vi "Handle getAll.vi"(8 "error in (no error)":errorcluster, 11 "Instrument.Transport in":refnum<class "Inst.Transport.lvclass">) -> (0 "error out":errorcluster, 2 "getAll":variant, 3 "Instrument.Transport out":refnum<class "Inst.Transport.lvclass">)   [LabVIEW 2019, in "Inst.Transport.lvclass"]
uses:
  Inst.Transport.lvclass
  Inst.Transport.lvclass/Inst.Transport.ctl
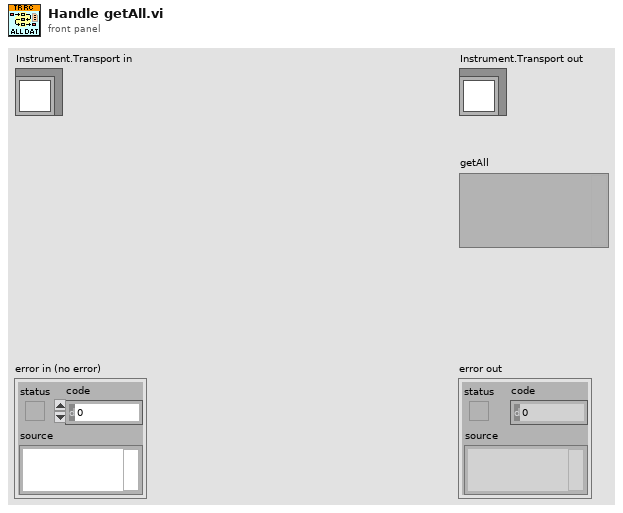
[diagram p1: front panel]
types:
  T1 = typedef "Inst.Transport.lvclass/Instrument.Transport.getAll--Cluster.ctl" = cluster{"Levy 1":dbl, "Logger SMO":dbl, "SMO Boolean":bool, "SMO String":string}
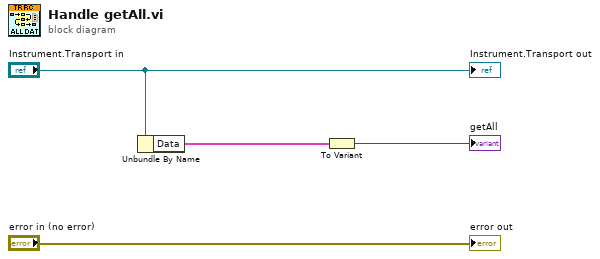
[diagram p0: block diagram]
diagram:
  n1 = Unbundle By Name("Instrument.Transport in") -> ("Data"=w1:T1)
  n2 = To Variant(anything=w1) -> (Variant=→"getAll":variant)
  "error out" <- "error in (no error)"
  "Instrument.Transport out" <- "Instrument.Transport in"
